vi "Cleanup.vi"(8 "error in (no error)":errorcluster, 11 "Editor in":refnum<class "Editor.lvclass">) -> (0 "error out":errorcluster)   [LabVIEW 2020, in "VolatusGUIEditor.lvlib" / "Editor.lvclass"]
uses:
  Editor.lvclass
  Editor.lvclass/Editor.ctl
  lv-oopanel/OOPanel/Manager/Manager.lvclass
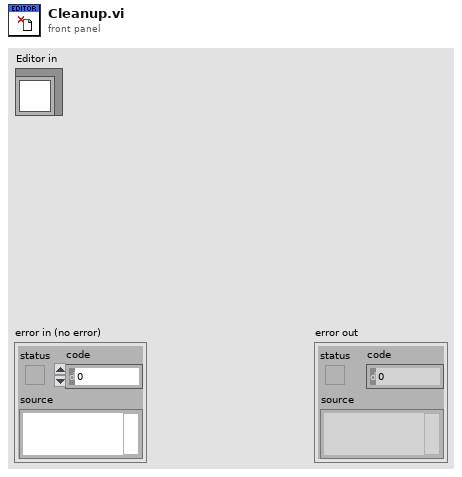
[diagram p1: front panel]
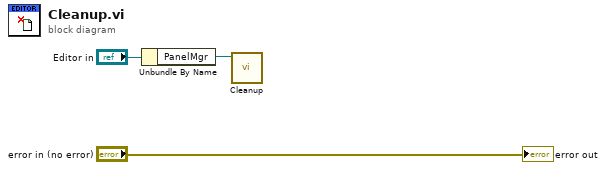
[diagram p0: block diagram]
diagram:
  n1 = Unbundle By Name("Editor in") -> ("PanelMgr"=w1:refnum<class "Manager.lvclass">)
  n2 = call "Cleanup.vi"("Manager in"=w1) -> ()  [unwired: 8 in, 3 out]
  "error out" <- "error in (no error)"
